vi "myTask.vi"(8 "error in (no error)":errorcluster, 10 "stopMechanism":refnum<class "ITaskStopMechanism.lvclass">, 11 "ITask in":refnum<class "ITask.lvclass">) -> (0 "error out":errorcluster, 3 "ITask out":refnum<class "ITask.lvclass">)   [LabVIEW 2023, in "Task_BoolUserEventStopMech.lvclass"]
doc: "_____________________________________\nTLC Daemon 1.0.0.2\nCopyright (c) 2026 Andrea Cadei"
uses:
  Task_BoolUserEventStopMech.lvclass
  ITask/ITask.lvclass
  ITaskStopMechanism/ITaskStopMechanism.lvclass
  BoolUserEventStopMech/BoolUserEventStopMechanism.lvclass
  C:/projects/TLC_Daemon/.source/ITask/ITask.lvclass
  Task_BoolUserEventStopMech.lvclass/Task_BoolUserEventStopMech.ctl
  Read description.vi
panel:
  out "loopCounter":i32 caption="Loop Counter"
  out "description":string
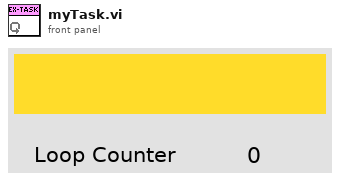
[diagram p1: front panel]
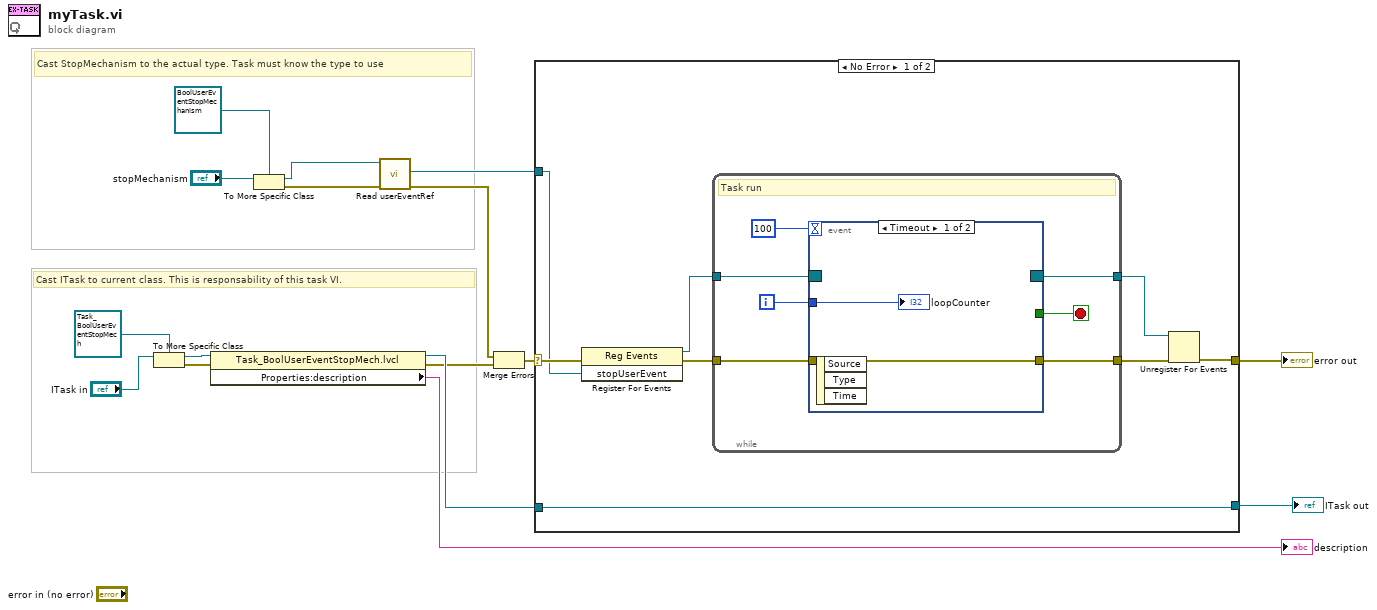
[diagram p0: block diagram]
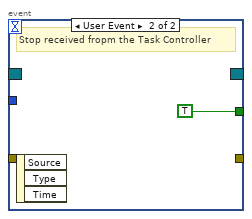
[diagram p2: hidden frame]
diagram:
  # "Cast ITask to current class. This is responsability of this task VI."
  # "Cast StopMechanism to the actual type. Task must know the type to use"
  n1 = To More Specific Class(target class=refnum<class "Task_BoolUserEventStopMech.lvclass"> refnum ("ExampleTask_StopNotifier.lvclass"), reference="ITask in") -> (specific class reference=w11:refnum<class "Task_BoolUserEventStopMech.lvclass">, error out=w12:errorcluster)  [unwired: 1 in]
  n2 = property class="Task_BoolUserEventStopMech.lvcl"(reference=w11, error in=w12) -> (reference out=w9:refnum<class "Task_BoolUserEventStopMech.lvclass">, error out=w7:errorcluster, "Properties:description"=→"description":string)
  n3 = To More Specific Class(target class=refnum<class "BoolUserEventStopMechanism.lvclass"> refnum ("TLC_Daemon.lvlib:NotifierStopMechanism.lvclass"), reference="stopMechanism") -> (specific class reference=w4:refnum<class "BoolUserEventStopMechanism.lvclass">, error out=w2:errorcluster)  [unwired: 1 in]
  n4 = call "Read userEventRef.vi"("error in (no error)"=w2, "BoolUserEventStopMechanism In"=w4) -> ("error out"=w1:errorcluster, "stopUserEvent"=w3:refnum<user-event>)  [unwired: 7 in, 1 out]
  n5 = Merge Errors(w1, w7) -> (w6:errorcluster)
  n6 = case shown="No Error" w6 {
    selector: w6 -> [w23 w36]
    tunnel: w3 -> [w21 _]
    tunnel: w9 -> [w24 w35]
    tunnel: [w24 w35] -> w8
    tunnel: [w18 w36] -> w5
    frame No Error {
      n7 = register-events(error in=w23, w21) -> (reference out=w20:refnum<event-registration>, error out=w22:errorcluster)  [unwired: 1 in]
      n8 = while {
        tunnel: w22 -> [w31]
        tunnel: [w30] -> w17
        tunnel: w20 -> [w27]
        tunnel: [w25] -> w19
        i -> [w29]
        stop <- w26 stop-if-true
        # "Task run"
        n9 = event shown="[0] Timeout" {
          selector: w27 -> [_ _]
          dyn-events: [_ _] -> w25
          timeout: 100 -> [_ _]
          tunnel: w31 -> [w33 _]
          tunnel: [w33 _] -> w30
          tunnel: w29 -> [w32 _]
          tunnel: [_ TRUE] -> w26
          event Timeout {
            n10 = event-data() -> ()  [unwired: 1 in, 3 out]
            "loopCounter" <- w32
          }
          event User Event {
            # "Stop received fropm the Task Controller"
            n11 = event-data() -> ()  [unwired: 1 in, 3 out]
          }
        }
      }
      n12 = Unregister For Events(event registration refnum=w19, error in=w17) -> (error out=w18:errorcluster)
    }
    frame Error {
    }
  }
  "error out" <- w5
  "ITask out" <- w8
